vi "PH_PSDBWriter.Wrap String Data.vi"(1 "Unit Array":string[](array[string]), 2 "Data Array":string[](array[string]), 3 "Name Array":string[](array[string]), 4 "Name Prefix":string) -> (0 "PSDB String Data Array":T1[](array[typedef]))   [LabVIEW 2014, in "PH_PSDBWriter.lvlib"]
doc: "This VI wrapes string data for the PSDB."
uses:
  PH_PSDBWriter.lvlib
  PH_PSDBWriter.String dataset.ctl
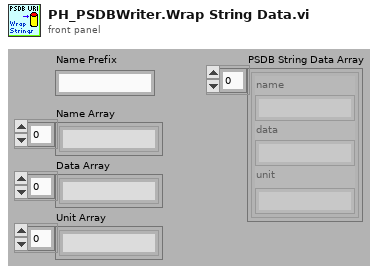
[diagram p1: front panel]
types:
  T1 = typedef "PH_PSDBWriter.lvlib/PH_PSDBWriter.String dataset.ctl" = cluster{"name":string, "data":string, "unit":string}
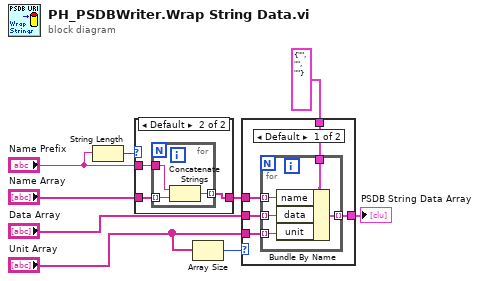
[diagram p0: block diagram]
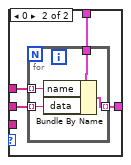
[diagram p2: hidden frame]
diagram:
  n1 = String Length(string="Name Prefix") -> (length=w2:i32)
  n2 = case shown="Default" w2 {
    tunnel: "Name Array" -> [w10 w13]
    tunnel: "Name Prefix" -> [_ w12]
    tunnel: [w10 w11] -> w3
    frame 0 {
    }
    frame Default {
      n3 = for {
        tunnel: w13 -> [w16] mode=indexing
        tunnel: w12 -> [w15]
        tunnel: [w14] -> w11 mode=indexing
        n4 = Concatenate Strings(w15, w16) -> (w14:string)
      }
    }
  }
  n5 = Array Size(array="Unit Array") -> (size(s)=w1:i32)
  n6 = case shown="Default" w1 {
    tunnel: [w21 w30] -> w9
    tunnel: T1 {"name"="", "data"="", "unit"=""} ("String data") -> [w20 w29]
    tunnel: "Data Array" -> [w19 w28]
    tunnel: "Unit Array" -> [w18 _]
    tunnel: w3 -> [w17 w27]
    frame Default {
      n7 = for {
        tunnel: w20 -> [w26]
        tunnel: w19 -> [w25] mode=indexing
        tunnel: w17 -> [w24] mode=indexing
        tunnel: [w23] -> w21 mode=indexing
        tunnel: w18 -> [w22] mode=indexing
        n8 = Bundle By Name(cluster=w26, "name"=w24, "data"=w25, "unit"=w22) -> (w23:T1)
      }
    }
    frame 0 {
      n9 = for {
        tunnel: w29 -> [w34]
        tunnel: w28 -> [w33] mode=indexing
        tunnel: w27 -> [w32] mode=indexing
        tunnel: [w31] -> w30 mode=indexing
        n10 = Bundle By Name(cluster=w34, "name"=w32, "data"=w33) -> (w31:T1)
      }
    }
  }
  "PSDB String Data Array" <- w9
